vi "IDSymmetry (SubVI).vi"(2 "Tolerance (%)":dbl, 3 "Values":dbl[](array[numeric]), 4 "Fit type":T2) -> (0 "Symmetry measure":dbl, 1 "Side of Tail":T1)   [LabVIEW 2016]
doc: "This VI assesses the symmetry around an extreme (max or min) of a set of values\nto determine if there are tails on the left or right hand sides of the exteme."
uses:
  Utils/Controls/All_Enums/Enum_TypeDef_ParabolaFitType.ctl
  Utils/Controls/All_Enums/Enum_TypeDef_Tails.ctl
panel:
  # "This VI assesses the symmetry around an extreme (max or min) of a set of values\nto determine if there are tails on the left or right hand sides of the exteme."
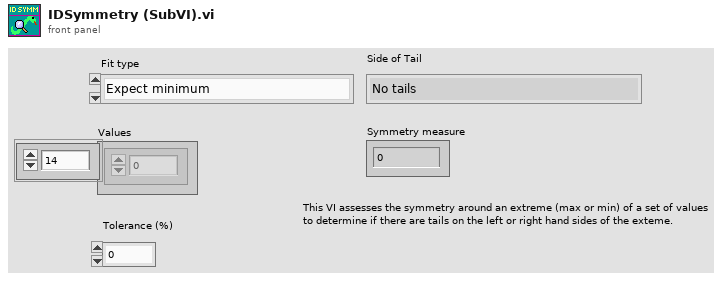
[diagram p1: front panel]
types:
  T1 = typedef "Enum_TypeDef_Tails.ctl" = enum16{"No tails", "Left tail", "Right tail"}
  T2 = typedef "Enum_TypeDef_ParabolaFitType.ctl" = enum16{"Expect minimum", "Expect maximum"}
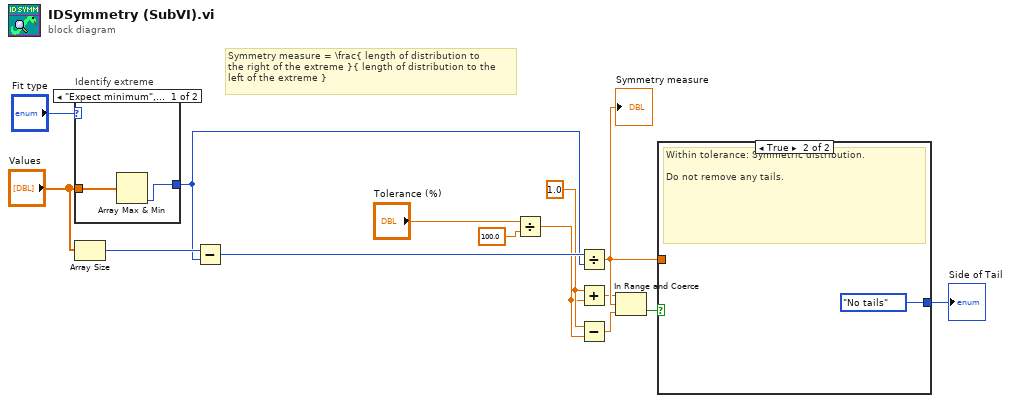
[diagram p0: block diagram]
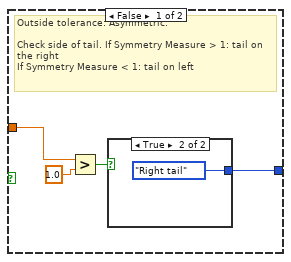
[diagram p2: hidden frame]
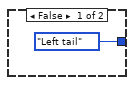
[diagram p3: hidden frame]
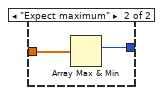
[diagram p4: hidden frame]
diagram:
  w3 = 1.0
  # "Symmetry measure = \\frac{ length of distribution to \nthe right of the extreme }{ length of distribution to the \nleft of the extreme }"
  n1 = case "Identify extreme" shown="\"Expect minimum\", Default" "Fit type" {
    tunnel: [w15 w18] -> w10
    tunnel: "Values" -> [w16 w17]
    frame "Expect minimum", Default {
      n2 = Array Max & Min(array=w16) -> (min index (indices)=w15:i32)  [unwired: 3 out]
    }
    frame "Expect maximum" {
      n3 = Array Max & Min(array=w17) -> (max index (indices)=w18:i32)  [unwired: 3 out]
    }
  }
  n4 = Array Size(array="Values") -> (size(s)=w13:i32)
  n5 = Subtract(x=w13, y=w10) -> (x-y=w11:i32)
  n6 = Divide(x="Tolerance (%)", y=100.0) -> (x/y=w2:dbl)
  n7 = Divide(x=w11, y=w10) -> (x/y=w7:dbl)
  "Symmetry measure" <- w7
  n8 = Add(x=w3, y=w2) -> (x+y=w4:dbl)
  n9 = Subtract(x=w3, y=w2) -> (x-y=w1:dbl)
  n10 = In Range and Coerce(upper limit=w4, x=w7, lower limit=w1) -> (In Range?=w9:bool)  [unwired: 1 out]
  n11 = case shown="True" w9 {
    tunnel: [w19 Enum_TypeDef_Tails."No tails" ("Side of Tail 2")] -> w8
    tunnel: w7 -> [w21 _]
    frame False {
      # "Outside tolerance: Asymmetric.\n\nCheck side of tail. If Symmetry Measure > 1: tail on the right\nIf Symmetry Measure < 1: tail on left"
      n12 = Greater?(x=w21, y=1.0) -> (0:w22:bool)
      n13 = case shown="True" w22 {
        tunnel: [Enum_TypeDef_Tails."Left tail" ("Side of Tail 2") Enum_TypeDef_Tails."Right tail" ("Side of Tail 2")] -> w19
        frame False {
        }
        frame True {
        }
      }
    }
    frame True {
      # "Within tolerance: Symmetric distribution.\n\nDo not remove any tails."
    }
  }
  "Side of Tail" <- w8
